vi "OpenMainConsole.vi"(3 "Baxter in":T2) -> (1 "Baxter out":T2)   [LabVIEW 2010]
uses:
  <userlib>/ROSforLV_0.1/ROS/Code/SubVIs/_ROSControl.ctl
  <userlib>/ROSforLV_0.1/ROS/Code/SubVIs/_ROSDirection.ctl
panel:
  out "Execution:State":T1(ring)
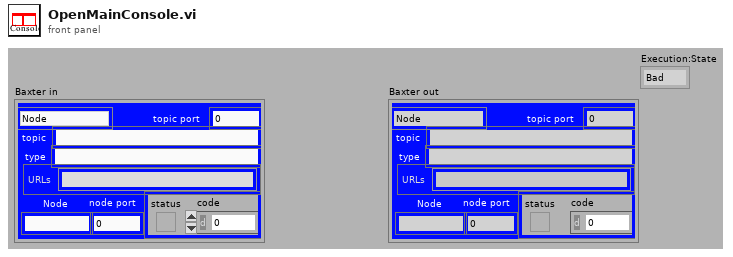
[diagram p1: front panel]
types:
  T1 = enum32{"Bad", "Idle", "Run top level", "Running"}
  T2 = typedef "_ROSControl.ctl" = cluster{"topic port":u16, "Node":string, "topic":string, "type":string, "node port":u32, "error ":errorcluster, "Direction":T3, "APIs":string[]}
  T3 = typedef "_ROSDirection.ctl" = enum16{"Node", "Publisher", "Subscriber", "Service Client"}
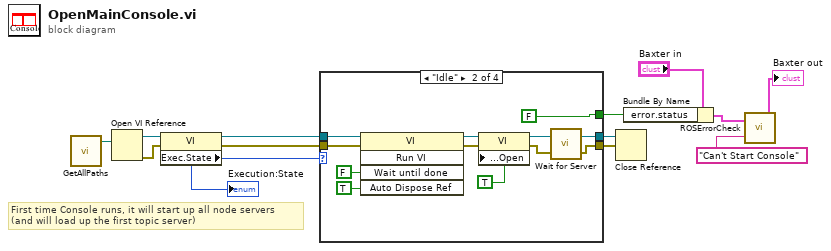
[diagram p0: block diagram]
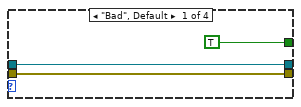
[diagram p2: hidden frame]
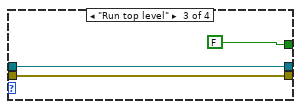
[diagram p3: hidden frame]
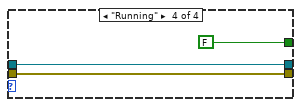
[diagram p4: hidden frame]
diagram:
  # "First time Console runs, it will start up all node servers\n(and will load up the first topic server)"
  n1 = call <userlib>:"GetAllPaths.vi"() -> ("Console Path"=w10:path)  [unwired: 1 in, 2 out]
  n2 = Open VI Reference(vi path=w10) -> (vi reference=w11:refnum<vi>, error out=w9:errorcluster)  [unwired: 5 in]
  n3 = property class="VI"(reference=w11, error in=w9) -> (error out=w8:errorcluster, "Exec.State"=w7:T1)  [unwired: 1 out]
  "Execution:State" <- w7
  n4 = case shown="\"Idle\"" w7 {
    tunnel: [w15 w17 w29 w32] -> w12
    tunnel: w11 -> [w15 w20 w29 w32]
    tunnel: [w14 w16 w28 w31] -> w6
    tunnel: w8 -> [w14 w25 w28 w31]
    tunnel: [TRUE ("Wait Until Done") FALSE ("Wait Until Done") FALSE ("Wait Until Done") FALSE ("Wait Until Done")] -> w2
    frame "Bad", Default {
    }
    frame "Idle" {
      n5 = invoke class="VI" method="Run VI"(reference=w20, error in=w25, "Wait until done"=FALSE ("Wait Until Done"), "Auto Dispose Ref"=TRUE ("Wait Until Done")) -> (reference out=w22:refnum<vi>, error out=w21:errorcluster)  [unwired: 1 in, 3 out]
      n6 = property class="VI"(reference=w22, error in=w21, "Front Panel.Open"=TRUE ("Wait Until Done")) -> (reference out=w18:refnum<vi>, error out=w19:errorcluster)
      n7 = call "Wait for Server.vi"("error in"=w19, "vi reference in"=w18) -> ("error out"=w16:errorcluster, "vi reference out"=w17:refnum<vi>)
    }
    frame "Run top level" {
    }
    frame "Running" {
    }
  }
  n8 = Close Reference(reference=w12, error in (no error)=w6) -> ()  [unwired: 1 out]
  n9 = Bundle By Name(cluster="Baxter in", "error.status"=w2) -> (w1:T2)
  n10 = call <userlib>:"ROSErrorCheck.vi"("message"="Can't Start Console", "ROS in"=w1) -> ("ROS out"=→"Baxter out":T2)  [unwired: 1 in]
